vi "serial_test.vi"() -> ()   [LabVIEW 2023]
uses:
  <vilib>/Instr/_visa.llb/VISA Configure Serial Port (Instr).vi
panel:
  out "Àã«×":string
  out "·Å«×":string
  in  "stop":bool
  out "return count":u32
  in  "¦ê¦C°ð":refnum<visa-resource-name>
  # "¢J"
  # "%"
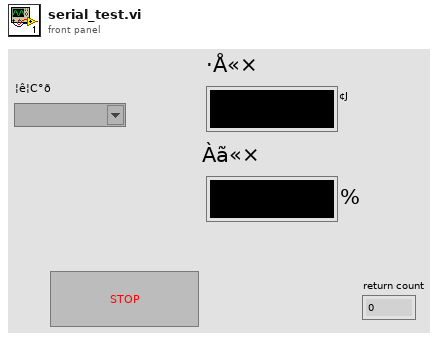
[diagram p1: front panel]
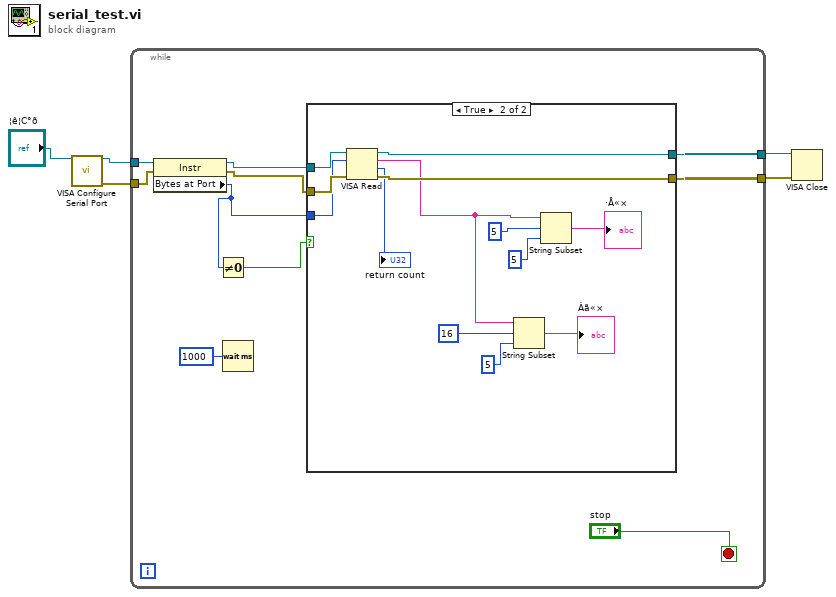
[diagram p0: block diagram]
diagram:
  n1 = call-poly "VISA Configure Serial Port"("VISA resource name"="¦ê¦C°ð") -> ("VISA resource name out"=w4:refnum<visa-resource-name>, "error out"=w3:errorcluster)  [unwired: 13 in]
  n2 = while {
    tunnel: w4 -> [w15]
    tunnel: w3 -> [w14]
    tunnel: [w9] -> w2
    tunnel: [w8] -> w1
    stop <- "stop" stop-if-true
    n3 = property class="Instr"(reference=w15, error in=w14) -> (reference out=w12:refnum<visa-resource-name>, error out=w11:errorcluster, "Bytes at Port"=w10:u32)
    n4 = Not Equal To 0?(x=w10) -> (x != 0?=w13:bool)
    n5 = Wait (ms)(milliseconds to wait=u32 1000) -> ()  [unwired: 1 out]
    n6 = case shown="True" w13 {
      tunnel: w12 -> [w17 w30]
      tunnel: w11 -> [w16 w29]
      tunnel: w10 -> [_ w28]
      tunnel: [w17 w27] -> w9
      tunnel: [w16 w26] -> w8
      frame False {
      }
      frame True {
        n7 = VISA Read(VISA resource name=w30, byte count=w28, error in (no error)=w29) -> (VISA resource name out=w27:refnum<visa-resource-name>, read buffer=w19:string, return count=→"return count":u32, error out=w26:errorcluster)
        n8 = String Subset(string=w19, offset (0)=16, length (rest)=5 ("length (rest)")) -> (substring=→"Àã«×":string)
        n9 = String Subset(string=w19, offset (0)=5, length (rest)=5 ("length (rest)")) -> (substring=→"·Å«×":string)
      }
    }
  }
  n10 = VISA Close(VISA resource name=w2, error in (no error)=w1) -> ()  [unwired: 1 out]
